vi "testteleop.vi"   [LabVIEW 2012, in "Test.lvrbt"]
uses:
  Test.lvrbt
  <vilib>/FTC/FTC Read Controller Packet.vi
  <vilib>/NXT/LegoClasses/BrickReference/BrickReference.lvclass
  <vilib>/NXT/Subs/LVHSConnector.ctl
  <vilib>/NXT/NXTIO Xnodes/NXTIOXNode/NXTIO.xnode
  <vilib>/NXT/NXTIO Xnodes/AddressXNode/NXTIOAddress.xnode
  <vilib>/FTC/FTC Interpret Motor Power From Left Y Axis.vi
  <vilib>/NXT/Hardware/Plugins/Tetrix DC Motor/TetrixDCMotorAddress.ctl
  <vilib>/FTC/FTC Interpret Motor Power From Right Y Axis.vi
  <vilib>/NXT/NXTIO Xnodes/NXTIONodeSubVIs/TETRIX IO Check Battery.vi
  <vilib>/NXT/NXTIO Xnodes/NXTIONodeSubVIs/TETRIX IO Stop DC Motors.vi
  <vilib>/NXT/NXTIO Xnodes/NXTIONodeSubVIs/TETRIX IO Move DC Motors.vi
panel:
  # "This VI was generated based on your configuration in the Remote Control Editor. You may modify the code as needed for your robot. To test this program for an FTC match, return to the Remote Control Editor, select the \"Run Program\" tab, and choose \"Teleop\"."
types:
  T1 = typedef "TetrixDCMotorAddress.ctl" = i32
  T2 = cluster{"TetrixDCMotor":T1, "TetrixDCMotor 2":T1}
  T3 = typedef "LVHSConnector.ctl" = refnum<class "BrickReference.lvclass">
  T4 = typedef "FTC ControllerState.ctl" = cluster{"Left X":i8, "Left Y":i8, "Right X":i8, "Right Y":i8, "Button Encoding 9-12":u8, "Button Encoding 1-8":u8, "POV":T5}
  T5 = typedef "FTC POVState.ctl" = i8
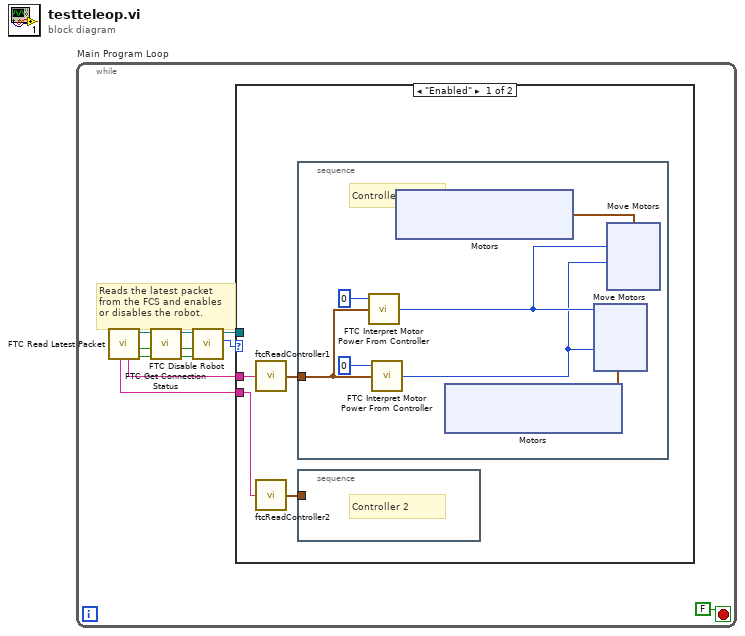
[diagram p0: block diagram]
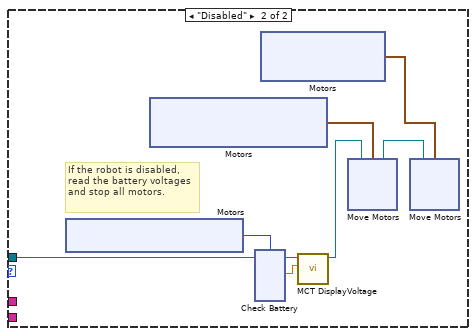
[diagram p2: hidden frame]
diagram:
  n1 = while "Main Program Loop" {
    stop <- FALSE stop-if-true
    # "Reads the latest packet\nfrom the FCS and enables\nor disables the robot."
    n2 = call <vilib>:"FTC Read Latest Packet.vi"() -> ("Packet Received?"=w8:bool, "Stopped?"=w5:bool, "NXT/EV3"=w7:T3, "Controller 1"=w10:string, "Controller 2"=w9:string)  [unwired: 6 in, 1 out]
    n3 = call <vilib>:"FTC Get Connection Status.vi"("Packet Received?"=w8, "Stopped?"=w5, "NXT/EV3"=w7) -> ("Online?"=w2:bool, "Stopped?"=w3:bool, "NXT/EV3"=w4:T3)  [unwired: 5 in]
    n4 = call <vilib>:"FTC Disable Robot.vi"("Online?"=w2, "Stopped?"=w3, "NXT/EV3"=w4) -> ("Enabled?"=w6:enum16{"Disabled", "Enabled"}, "NXT/EV3"=w1:T3)  [unwired: 3 in]
    n5 = case "disableCase" shown="\"Enabled\"" w6 {
      tunnel: w10 -> [w15 _]
      tunnel: w9 -> [w14 _]
      tunnel: w1 -> [_ w48]
      frame "Enabled" {
        n6 = call "ftcReadController1"("Packet"=w15) -> ("Controller State"=w13:T4)  [unwired: 4 in]
        n7 = call "ftcReadController2"("Packet"=w14) -> ("Controller State"=w12:T4)  [unwired: 4 in]
        n8 = stacked-sequence "controller1Actions" {
          tunnel: w13 -> [w22]
          frame #0 {
            # "Controller 1"
            n9 = call-poly <vilib>:"FTC Interpret Motor Power From Controller.vi"("Controller State"=w22, "Power Level (50)"=i8 0) -> ("Power"=w17:i8)  [unwired: 1 in]
            n10 = call-poly <vilib>:"FTC Interpret Motor Power From Controller.vi"("Controller State"=w22, "Power Level (50)"=i8 0) -> ("Power"=w16:i8)  [unwired: 1 in]
            n11 = xnode ("Motors")() -> ("Motor"=w20:cluster{"TetrixDCMotor":T1, "TetrixDCMotor":T1})
            n12 = xnode ("Motors")() -> ("Motor"=w18:cluster{"TetrixDCMotor":T1, "TetrixDCMotor":T1})
            n13 = xnode ("Move Motors")("Power/Speed 2"=w16, "Power/Speed 1"=w17, "Motors"=w18) -> ()  [unwired: 1 in, 1 out]
            n14 = xnode ("Move Motors")("Power/Speed 2"=w16, "Power/Speed 1"=w17, "Motors"=w20) -> ()  [unwired: 1 in, 1 out]
          }
        }
        n15 = stacked-sequence "controller2Actions" {
          tunnel: w12 -> [_]
          frame #0 {
            # "Controller 2"
          }
        }
      }
      frame "Disabled" {
        # "If the robot is disabled, read the battery voltages and stop all motors."
        n16 = xnode ("Motors")() -> ("Motor"=w47:T1)
        n17 = xnode "Motors"() -> ("Motor"=w44:cluster{"TetrixDCMotor":T1, "TetrixDCMotor":T1})
        n18 = xnode ("Check Battery")("Motors"=w47, "NXT/EV3"=w48) -> ("Voltage 1"=w46:sgl, "NXT/EV3"=w45:T3)
        n19 = xnode "Motors"() -> ("Motor"=w42:cluster{"TetrixDCMotor":T1, "TetrixDCMotor":T1})
        n20 = call <vilib>:"MCT DisplayVoltage.vi"("Motor Voltage"=w46, "NXT/EV3"=w45) -> ("NXT/EV3"=w43:T3)  [unwired: 9 in]
        n21 = xnode "Move Motors"("Motors"=w44, "NXT/EV3"=w43) -> ("NXT/EV3"=w41:T3)
        n22 = xnode "Move Motors"("Motors"=w42, "NXT/EV3"=w41) -> ()  [unwired: 1 out]
      }
    }
  }
